vi "Ex1_Arithmetic_Operations.vi"() -> ()   [LabVIEW 2024]
panel:
  out "Result":dbl
  in  "Operand 2":dbl
  in  "Operand 1":dbl
  out "Result":dbl
  in  "Operand 2":dbl
  in  "Operand 1":dbl
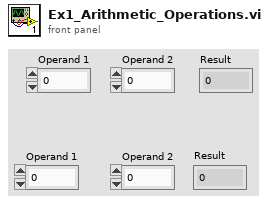
[diagram p1: front panel]
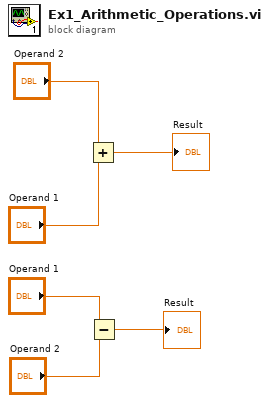
[diagram p0: block diagram]
diagram:
  n1 = Add(x="Operand 2", y="Operand 1") -> (x+y=→"Result":dbl)
  n2 = Subtract(x="Operand 1", y="Operand 2") -> (x-y=→"Result":dbl)
